vi "test_ClientFGV_RecreateClientTwice_ClientCreatedTwice.vi"(8 "error in":errorcluster) -> (0 "error out":errorcluster, 2 "result":string, 3 "pass":bool)   [LabVIEW 2020, in "MeasurementServerTests.lvlib" / "gRPC Utilities Tests.lvlib"]
uses:
  gRPC Utilities Tests.lvlib
  Runtime/MeasurementLink gRPC Utilities/gRPC Client Pool Helpers/Action.ctl
  <vilib>/gRPC/LabVIEW gRPC Library/Shared/grpcId.ctl
  Runtime/MeasurementLink gRPC Utilities/MeasurementLink gRPC Utilities.lvlib
  <vilib>/gRPC/LabVIEW gRPC Library/grpc-lvsupport-release.lvlib
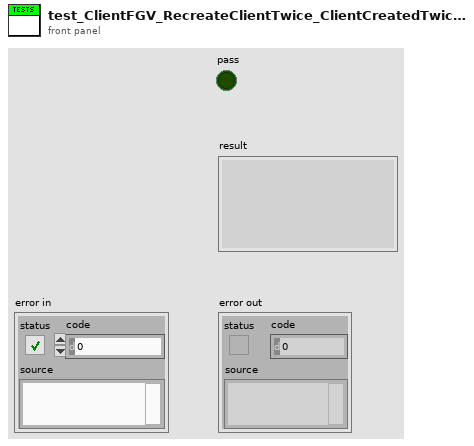
[diagram p1: front panel]
types:
  T1 = typedef "grpc-lvsupport-release.lvlib/grpcId.ctl" = u64
  T2 = typedef "MeasurementLink gRPC Utilities.lvlib/Action.ctl" = enum16{"Get Client", "Recreate Client"}
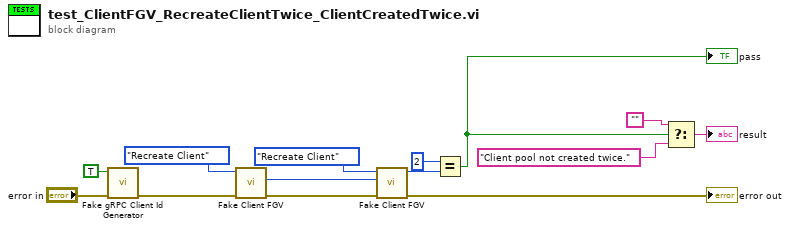
[diagram p0: block diagram]
diagram:
  n1 = call "Fake gRPC Client Id Generator.vi"("error in"="error in", "reset generator"=TRUE) -> ("error out"=w6:errorcluster)  [unwired: 8 in, 1 out]
  n2 = call "Fake Client FGV.vi"("error in"=w6, "action"=Action."Recreate Client") -> ("error out"=w8:errorcluster, "unique id out"=w1:u64)  [unwired: 7 in, 1 out]
  n3 = call "Fake Client FGV.vi"("error in"=w8, "unique id in"=w1, "action"=Action."Recreate Client") -> ("error out"=→"error out":errorcluster, "grpc client id"=w4:T1)  [unwired: 6 in, 1 out]
  n4 = Equal?(x=T1 2, y=w4) -> (x = y?=w2:bool)
  "pass" <- w2
  n5 = Select(t="", s=w2, f="Client pool not created twice.") -> (s? t:f=→"result":string)
